vi "Parse Bitfile EST Clusters.vi"(8 "error in (no error)":errorcluster, 11 "bitfile path":path) -> (0 "error out":errorcluster, 1 "version":string, 2 "EPS IP LUT":variant, 3 "valid bitfile":bool, 4 "EST version enum":T1)   [LabVIEW 2013, in "Engine Simulation Toolkit System Explorer.lvlib"]
uses:
  Engine Simulation Toolkit System Explorer.lvlib
  Shared/Bitfile EST Version.ctl
  Shared/Properties.vi
  Shared/Engine Simulation Toolkit Shared.lvlib
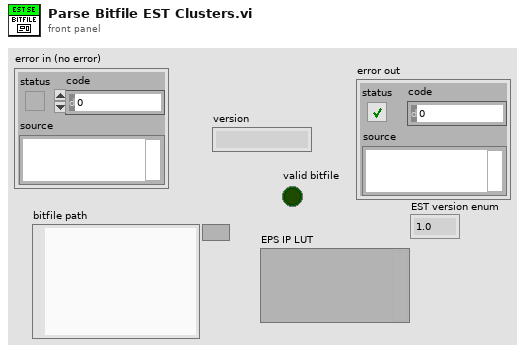
[diagram p1: front panel]
types:
  T1 = typedef "Engine Simulation Toolkit Shared.lvlib/Bitfile EST Version.ctl" = enum16{"1.0", "1.1", "1.2", "1.3"}
  T2 = typedef "niFpgaBitfileStructure_VI.ctl" = cluster{"Name":string, "RegisterMap":T3[], "Icon":T8}
  T3 = typedef "nirviControlStructure.ctl" = cluster{"Name":string, "Hidden":bool, "Indicator":bool, "Flattened Type":string, "Grouping":cluster{"Grouped":bool, "Member Names":string[], "Member IDs":u32[]}, "Address":u32, "Size":u32, "Class":u32, "Internal":bool, "Typedef":T4, "ID":u32, "Bidirectional":bool, "Synchronous":bool, "Mechanical Action":T5, "Sub Controls":T6[], "Access May Timeout":bool, "Register Node":bool}
  T4 = typedef "nirviTypdefDescription.ctl" = cluster{"Typedef":bool, "Path":path}
  T5 = typedef "nirviMechanicalAction.ctl" = enum8{"Switch When Pressed", "Switch When Released", "Switch Until Released", "Latch When Pressed", "Latch When Released", "Latch Until Released"}
  T6 = typedef "nirviSubControlStructure.ctl" = cluster{"Name":string, "flattened Type":string, "Cluster Information":T7, "Typedef":T4}
  T7 = typedef "nirviClusterElementControl.ctl" = cluster{"Name Hierarchy":string[], "Item Order":u32[]}
  T8 = typedef "imagedata.ctl" = cluster{"image type":i32, "image depth":i32, "image":u8[], "mask":u8[], "colors":u32[], "Rectangle":cluster{"left":i16, "top":i16, "right":i16, "bottom":i16}}
  T9 = typedef "Engine Simulation Toolkit Shared.lvlib/IP Interface Enum.ctl" = enum16{"APU Settings", "APU Shared Settings", "APU Output", "APU Input", "Analog Replay Settings", "Analog Replay Load Input", "Analog Replay Input", "ETiming Capture Output", "ETiming Meas Settings", "ETiming Meas Output", "Digital PatGen Settings", "Digital PatGen Input", "Digital PatGen Load Input", "Knock Sensor Input", "Knock Sensor Settings", "Knock Cyl Input", "Knock Cyl Settings", "Dir Speed Input", "Dir Speed Settings", "Dir Speed Load Input", "APU Go"}
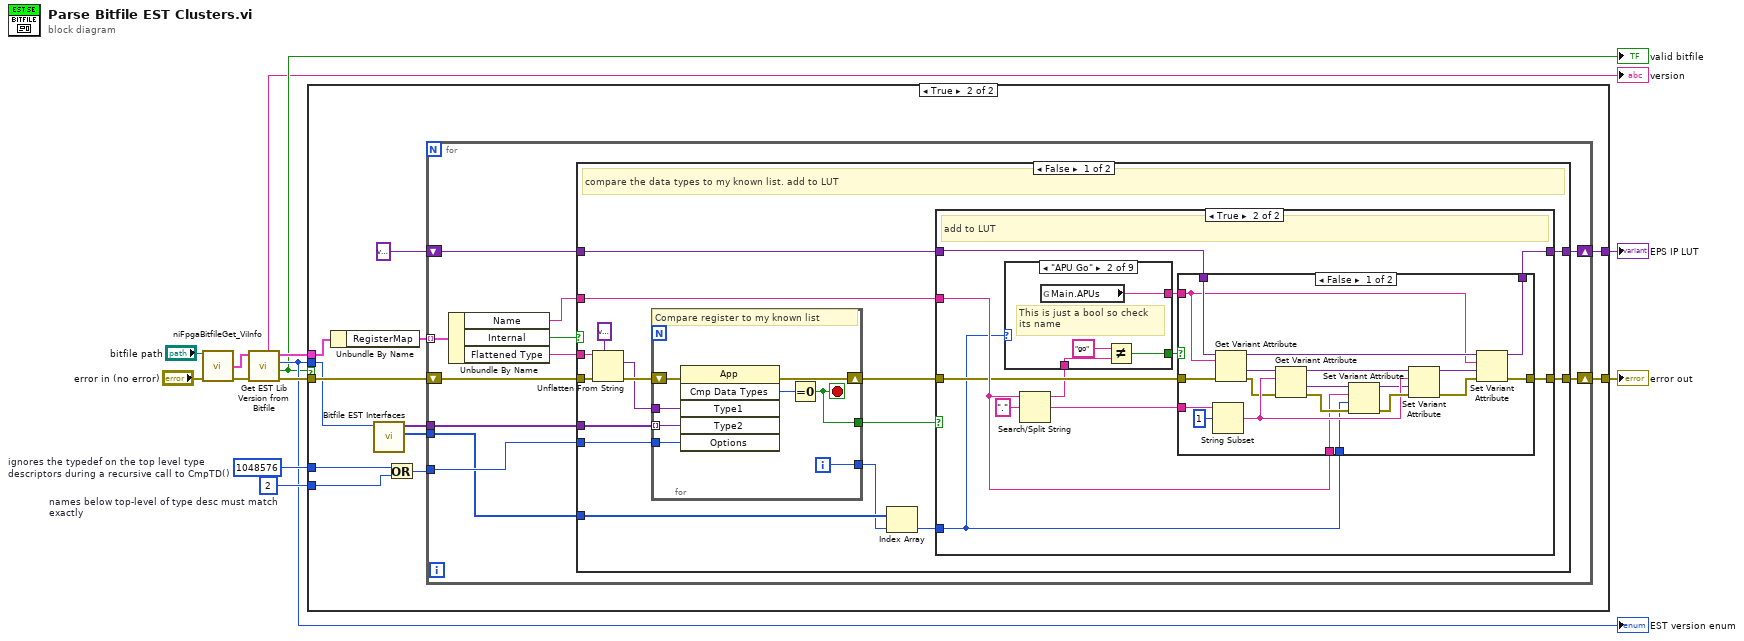
[diagram p0: block diagram]
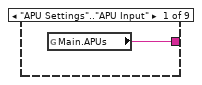
[diagram p5: hidden frame]
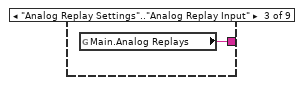
[diagram p6: hidden frame]
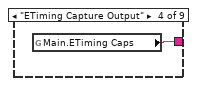
[diagram p7: hidden frame]
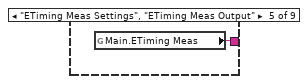
[diagram p8: hidden frame]
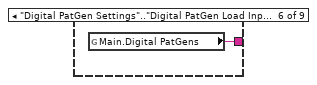
[diagram p9: hidden frame]
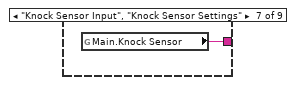
[diagram p10: hidden frame]
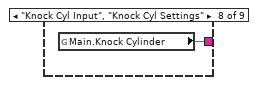
[diagram p11: hidden frame]
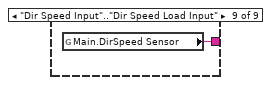
[diagram p12: hidden frame]
diagram:
  w10 = 2  # names below top-level of type desc must match exactly
  w11 = 1048576  # ignores the typedef on the top level type descriptors during a recursive call to CmpTD()
  n1 = call <vilib>:"niFpgaBitfileGet_ViInfo.vi"("bitfile path"="bitfile path", "error in (no error)"="error in (no error)") -> ("vi info"=w5:T2, "error out"=w12:errorcluster)  [unwired: 1 in, 11 out]
  n2 = call "Get EST Lib Version from Bitfile.vi"("error in (no error)"=w12, "vi info"=w5) -> ("error out"=w6:errorcluster, "valid bitfile"=w2:bool, "EST version enum"=w3:T1, "vi info dup"=w4:T2, "EST version string"=→"version":string)  [unwired: 5 in]
  "valid bitfile" <- w2
  "EST version enum" <- w3
  n3 = case shown="True" w2 {
    tunnel: w11 -> [_ w25]
    tunnel: w10 -> [_ w23]
    tunnel: [w14 w20] -> w9
    tunnel: [_ w18] -> w7
    tunnel: w6 -> [w14 w17]
    tunnel: w4 -> [_ w16]
    tunnel: w3 -> [_ w15]
    frame False {
    }
    frame True {
      n4 = Unbundle By Name(w16) -> ("RegisterMap"=w26:T3[])
      n5 = call "Bitfile EST Interfaces.vi"("Version"=w15) -> ("IP Types"=w21:T9[], "IP Interface"=w22:variant[])  [unwired: 9 in]
      n6 = Or(x=w25, y=w23) -> (x .or. y?=w24:i32)
      n7 = for {
        shift-right: [w37] -> w20
        shift-left: w17 -> [w34]
        tunnel: w26 -> [w36] mode=indexing
        tunnel: w24 -> [w31]
        tunnel: w22 -> [w30]
        tunnel: w21 -> [w29]
        shift-right: [w27] -> w18
        shift-left: variant ("Variant") -> [w28]
        n8 = Unbundle By Name(w36) -> ("Name"=w35:string, "Internal"=w32:bool, "Flattened Type"=w33:string)
        n9 = case shown="False" w32 {
          tunnel: [w43 w110] -> w37
          tunnel: w35 -> [w42 _]
          tunnel: w34 -> [w52 w110]
          tunnel: w33 -> [w50 _]
          tunnel: w31 -> [w48 _]
          tunnel: w30 -> [w47 _]
          tunnel: w29 -> [w46 _]
          tunnel: w28 -> [w45 w109]
          tunnel: [w44 w109] -> w27
          frame False {
            # "compare the data types to my known list. add to LUT"
            n10 = Unflatten From String(type=variant ("Variant"), binary string=w50, error in (no error)=w52) -> (value=w49:variant, error out=w53:errorcluster)  [unwired: 3 out]
            n11 = for {
              shift-right: [w107] -> w38
              shift-left: w53 -> [w108]
              tunnel: w49 -> [w105]
              tunnel: w47 -> [w104] mode=indexing
              tunnel: [w103] -> w39
              tunnel: [w102] -> w41
              tunnel: w48 -> [w101]
              i -> [w102]
              stop <- w103 stop-if-true
              # "Compare register to my known list"
              n12 = invoke class="App" method="Cmp Data Types"(error in=w108, "Type1"=w105, "Type2"=w104, "Options"=w101) -> (error out=w107:errorcluster, "Compare Data Types"=w106:i32)  [unwired: 2 in, 4 out]
              n13 = Equal To 0?(x=w106) -> (x = 0?=w103:bool)
            }
            n14 = Index Array(array=w46, index=w41) -> (element=w40:T9)
            n15 = case shown="True" w39 {
              tunnel: w40 -> [_ w58]
              tunnel: w45 -> [w54 w62]
              tunnel: [w54 w60] -> w44
              tunnel: w42 -> [_ w64]
              tunnel: [w55 w61] -> w43
              tunnel: w38 -> [w55 w63]
              frame False {
              }
              frame True {
                # "add to LUT"
                n16 = Search/Split String(string=w64, search string/char (-)=".") -> (substring before match=w57:string, match + rest of string=w65:string)  [unwired: 1 in, 1 out]
                n17 = case shown="\"APU Go\"" w58 {
                  tunnel: [w89 w93 w94 w95 w96 w97 w98 w99 w100] -> w59
                  tunnel: w57 -> [_ w92 _ _ _ _ _ _ _]
                  tunnel: [_ w90 _ _ _ _ _ _ _] -> w56
                  frame "APU Settings".."APU Input" {
                    n18 = global read "Properties.vi" "Main.APUs"() -> (w89:string)
                  }
                  frame "APU Go" {
                    # "This is just a bool so check its name"
                    n19 = global read "Properties.vi" "Main.APUs"() -> (w93:string)
                    n20 = Not Equal?(x="go", y=w92) -> (x != y?=w90:bool)
                  }
                  frame "Analog Replay Settings".."Analog Replay Input" {
                    n21 = global read "Properties.vi" "Main.Analog Replays"() -> (w94:string)
                  }
                  frame "ETiming Capture Output" {
                    n22 = global read "Properties.vi" "Main.ETiming Caps"() -> (w95:string)
                  }
                  frame "ETiming Meas Settings", "ETiming Meas Output" {
                    n23 = global read "Properties.vi" "Main.ETiming Meas"() -> (w96:string)
                  }
                  frame "Digital PatGen Settings".."Digital PatGen Load Input" {
                    n24 = global read "Properties.vi" "Main.Digital PatGens"() -> (w97:string)
                  }
                  frame "Knock Sensor Input", "Knock Sensor Settings" {
                    n25 = global read "Properties.vi" "Main.Knock Sensor"() -> (w98:string)
                  }
                  frame "Knock Cyl Input", "Knock Cyl Settings" {
                    n26 = global read "Properties.vi" "Main.Knock Cylinder"() -> (w99:string)
                  }
                  frame "Dir Speed Input".."Dir Speed Load Input" {
                    n27 = global read "Properties.vi" "Main.DirSpeed Sensor"() -> (w100:string)
                  }
                }
                n28 = case shown="False" w56 {
                  tunnel: w65 -> [w86 _]
                  tunnel: w64 -> [w78 _]
                  tunnel: w63 -> [w76 w88]
                  tunnel: w62 -> [w73 w87]
                  tunnel: [w72 w88] -> w61
                  tunnel: [w70 w87] -> w60
                  tunnel: w59 -> [w68 _]
                  tunnel: w58 -> [w67 _]
                  frame False {
                    n29 = String Subset(string=w86, offset (0)=1) -> (substring=w81:string)  [unwired: 1 in]
                    n30 = Get Variant Attribute(Variant=w73, name=w68, error in=w76) -> (duplicate Variant=w71:variant, value=w74:variant, error out=w75:errorcluster)  [unwired: 1 in, 1 out]
                    n31 = Get Variant Attribute(Variant=w74, name=w81, error in=w75) -> (duplicate Variant=w79:variant, value=w83:variant, error out=w84:errorcluster)  [unwired: 1 in, 1 out]
                    n32 = Set Variant Attribute(Variant=w83, name=w78, value=w67, error in=w84) -> (Variant out=w80:variant, error out=w82:errorcluster)  [unwired: 1 out]
                    n33 = Set Variant Attribute(Variant=w79, name=w81, value=w80, error in=w82) -> (Variant out=w69:variant, error out=w77:errorcluster)  [unwired: 1 out]
                    n34 = Set Variant Attribute(Variant=w71, name=w68, value=w69, error in=w77) -> (Variant out=w70:variant, error out=w72:errorcluster)  [unwired: 1 out]
                  }
                  frame True {
                  }
                }
              }
            }
          }
          frame True {
            # "avoid internal registers. They don't have a type and users didnt make them anyway"
          }
        }
      }
    }
  }
  "error out" <- w9
  "EPS IP LUT" <- w7
